vi "02lee_config_equipos.vi"(1 "Config Equipos ent":T1(array[cluster]) {"Ref PD 2" max=10000 step=1; "Med Princ" items=["1", "2", "3", "4", "5", "6", "7", "8", "9", "10", "11", "12", "13", "14", "15", "16", "17", "18", "19", "20", "21", "22", "23", "24", "25", "26", "27", "28", "29", "30", "31", "32"]}, 2 "Equipo Nº":i32, 3 "exe path":string) -> (0 "Config Equipos sal":T1(array[cluster]) {"Ref PD 2" max=10000 step=1; "Med Princ" items=["1", "2", "3", "4", "5", "6", "7", "8", "9", "10", "11", "12", "13", "14", "15", "16", "17", "18", "19", "20", "21", "22", "23", "24", "25", "26", "27", "28", "29", "30", "31", "32"]})   [LabVIEW 2010]
uses:
  <vilib>/Utility/file.llb/Write To Spreadsheet File (string).vi
  <vilib>/Utility/file.llb/Write To Spreadsheet File (I64).vi
  <vilib>/Utility/file.llb/Read From Spreadsheet File (string).vi
  <vilib>/Utility/file.llb/Read From Spreadsheet File (I64).vi
panel:
  out "error out":errorcluster
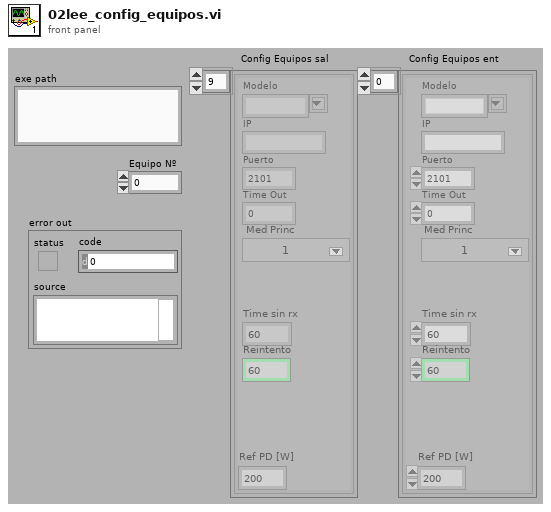
[diagram p1: front panel]
types:
  T1 = cluster{"Modelo":string, "IP":string, "Puerto":u16, "Time Out":u16, "Med Princ":u16, "Time sin rx":u16, "Reintento":u16, "Ref PD 2":u16}[]
  T2 = cluster{"Modelo":string, "IP":string, "Puerto":u16, "Time out":u16, "Med princ":u16, "Barrido":u16, "Time sin Rx":u16, "tam Reg":u16}
  T3 = cluster{"Puerto":u16, "Time out":u16, "Med princ":u16, "Barrido":u16, "Time sin Rx":u16, "tam Reg":u16}
  T4 = cluster{"[0]":u16, "[1]":u16, "[2]":u16, "[3]":u16, "[4]":u16, "[5]":u16}
  T5 = cluster{"first row[0]":string, "first row[1]":string}
  T6 = cluster{"first row[0]":string, "first row[1]":string, "[0]":u16, "[1]":u16, "[2]":u16, "[3]":u16, "[4]":u16, "[5]":u16}
  T7 = cluster{"Modelo":string, "IP":string, "Puerto":u16, "Time Out":u16, "Med Princ":u16, "Time sin rx":u16, "Reintento":u16, "Ref PD 2":u16}
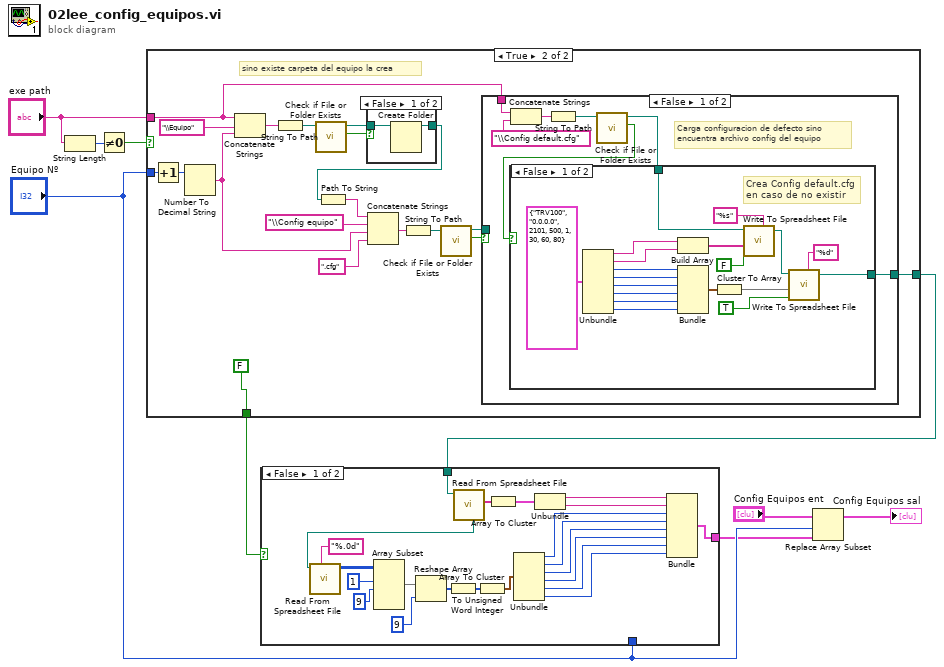
[diagram p0: block diagram]
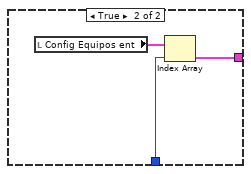
[diagram p2: hidden frame]
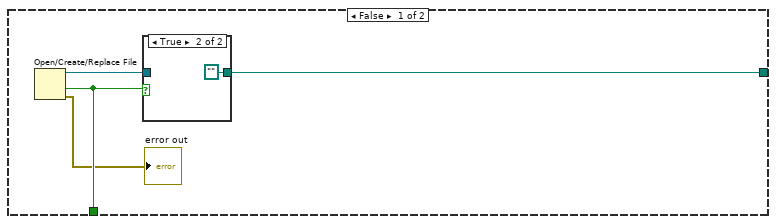
[diagram p3: hidden frame]
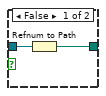
[diagram p4: hidden frame]
diagram:
  n1 = String Length(string="exe path") -> (length=w8:i32)
  n2 = Not Equal To 0?(x=w8) -> (x != 0?=w7:bool)
  n3 = case shown="True" w7 {
    tunnel: "Equipo Nº" -> [_ w32]
    tunnel: "exe path" -> [_ w18]
    tunnel: [w12 w17] -> w6
    tunnel: [w11 FALSE ("cancelled")] -> w5
    frame False {
      n4 = Open/Create/Replace File() -> (refnum out=w13:refnum<file>, cancelled=w11:bool, error out=→"error out":errorcluster)  [unwired: 1 in, 5 out]
      n5 = case shown="True" w11 {
        tunnel: w13 -> [w15 _]
        tunnel: [w14 path ""] -> w12
        frame False {
          n6 = Refnum to Path(1:w15) -> (0:w14:path)
        }
        frame True {
        }
      }
    }
    frame True {
      # "sino existe carpeta del equipo la crea"
      n7 = Increment(x=w32) -> (x+1=w31:i32)
      n8 = Number To Decimal String(number=w31) -> (decimal integer string=w25:string)  [unwired: 1 out]
      n9 = Concatenate Strings(w18, "\\Equipo" ("replace string (\"\")"), w25) -> (w27:string)
      n10 = String To Path(string=w27) -> (path=w28:path)
      n11 = call <vilib>:"Check if File or Folder Exists.vi"("path"=w28) -> ("file or folder exists?"=w29:bool, "dup path"=w30:path)  [unwired: 1 in, 8 out]
      n12 = case shown="False" w29 {
        tunnel: [w65 w66] -> w22
        tunnel: w30 -> [w64 w66]
        frame False {
          n13 = Create Folder(path (use dialog)=w64) -> (created path=w65:path)  [unwired: 1 in, 3 out]
        }
        frame True {
        }
      }
      n14 = Path To String(path=w22) -> (string=w21:string)
      n15 = Concatenate Strings(w21, "\\Config equipo" ("replace string (\"\")"), w25, ".cfg" ("replace string (\"\")")) -> (w23:string)
      n16 = String To Path(string=w23) -> (path=w33:path)
      n17 = call <vilib>:"Check if File or Folder Exists.vi"("path"=w33) -> ("file or folder exists?"=w34:bool, "dup path"=w35:path)  [unwired: 1 in, 8 out]
      n18 = case shown="False" w34 {
        tunnel: w35 -> [_ w63]
        tunnel: [w39 w63] -> w17
        tunnel: w18 -> [w42 _]
        frame False {
          # "Carga configuracion de defecto sino\nencuentra archivo config del equipo"
          n19 = Concatenate Strings(w42, "\\Config default.cfg" ("replace string (\"\")")) -> (w41:string)
          n20 = String To Path(string=w41) -> (path=w37:path)
          n21 = call <vilib>:"Check if File or Folder Exists.vi"("path"=w37) -> ("file or folder exists?"=w38:bool, "dup path"=w36:path)  [unwired: 1 in, 8 out]
          n22 = case shown="False" w38 {
            tunnel: [w43 w62] -> w39
            tunnel: w36 -> [w44 w62]
            frame False {
              # "Crea Config default.cfg\nen caso de no existir"
              n23 = Unbundle(T2 {"Modelo"="TRV100", "IP"="0.0.0.0", "Puerto"=2101, "Time out"=500, "Med princ"=1, "Barrido"=30, "Time sin Rx"=60, "tam Reg"=80} ("Config equipo")) -> ("Modelo"=w61:string, "IP"=w60:string, "Puerto"=w59:u16, "Time out"=w58:u16, "Med princ"=w57:u16, "Barrido"=w56:u16, "Time sin Rx"=w55:u16, "tam Reg"=w54:u16)
              n24 = Build Array(w61, w60) -> (w51:string[])
              n25 = Bundle("Puerto"=w59, "Time out"=w58, "Med princ"=w57, "Barrido"=w56, "Time sin Rx"=w55, "tam Reg"=w54) -> (w52:T3)  [unwired: 1 out]
              n26 = Cluster To Array(cluster=w52) -> (array=w50:u16[])
              n27 = call-poly <vilib>:"Write To Spreadsheet File.vi"("format (%s)"="%s" ("format (%d)"), "append to file? (new file:F)"=FALSE, "1D data"=w51, "file path (dialog if empty)"=w44) -> ("new file path (Not A Path if cancelled)"=w47:path)  [unwired: 2 in, 2 out]
              n28 = call-poly <vilib>:"Write To Spreadsheet File.vi"("format (%d)"="%d", "append to file? (new file:F)"=TRUE, "1D data"=w50, "file path (dialog if empty)"=w47) -> ("new file path (Not A Path if cancelled)"=w43:path)  [unwired: 2 in, 2 out]
            }
            frame True {
            }
          }
        }
        frame True {
        }
      }
    }
  }
  n29 = case shown="False" w5 {
    tunnel: w6 -> [w67 _]
    tunnel: "Equipo Nº" -> [_ w90]
    tunnel: [w70 w89] -> w3
    frame False {
      n30 = call-poly <vilib>:"Read From Spreadsheet File.vi"("file path (dialog if empty)"=w67) -> ("first row"=w83:string[], "new file path (Not A Path if cancelled)"=w71:path)  [unwired: 3 in, 6 out]
      n31 = call-poly <vilib>:"Read From Spreadsheet File.vi"("format (%d)"="%.0d", "file path (dialog if empty)"=w71) -> ("all rows"=w76:i64[][])  [unwired: 2 in, 7 out]
      n32 = Array Subset(array=w76, index (row)=1 ("index"), length (row)=9 ("length")) -> (w79:i64[][])  [unwired: 2 in]
      n33 = Reshape Array(w79, 9 ("dimension size")) -> (w74:i64[])
      n34 = To Unsigned Word Integer(number=w74) -> (unsigned 16bit integer=w75:u16[])
      n35 = Array To Cluster(array=w75) -> (cluster=w78:T4)
      n36 = Array To Cluster(array=w83) -> (cluster=w84:T5)
      n37 = Unbundle(w78) -> ("[0]"=w73:u16, "[1]"=w72:u16, "[2]"=w85:u16, "[3]"=w86:u16, "[4]"=w87:u16, "[5]"=w88:u16)
      n38 = Unbundle(w84) -> ("first row[0]"=w68:string, "first row[1]"=w69:string)
      n39 = Bundle("first row[0]"=w68, "first row[1]"=w69, "[0]"=w73, "[1]"=w72, "[2]"=w85, "[3]"=w86, "[4]"=w87, "[5]"=w88) -> (w70:T6)  [unwired: 1 out]
    }
    frame True {
      n40 = local read "Config Equipos ent"() -> (w91:T1)
      n41 = Index Array(array=w91, index=w90) -> (element=w89:T7)
    }
  }
  n42 = Replace Array Subset(array="Config Equipos ent", new element=w3, index="Equipo Nº") -> (→"Config Equipos sal":T1)
